vi "Mapping_GBL.vi"() -> ()   [LabVIEW 2017]
uses:
  Ctl/Current_Position.ctl
panel:
  in  "LaserScan_angle_min":dbl
  in  "LaserScan_angles_increment":dbl
  in  "LaserScanangles[]":dbl[](array[numeric])
  in  "LaserScandistance[]":dbl[](array[numeric])
  in  "Current_Position":T1
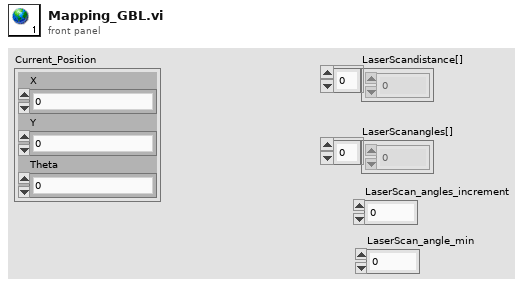
[diagram p1: front panel]
types:
  T1 = typedef "Current_Position.ctl" = cluster{"X":dbl, "Y":dbl, "Theta":dbl}
diagram:
